vi "ContinuosSoundEntry.vi"() -> ()   [LabVIEW 2015]
uses:
  <vilib>/sound2/lvsound2.llb/Sound Data Format.ctl
  <vilib>/sound2/lvsound2.llb/Sampling Mode.ctl
  <vilib>/sound2/lvsound2.llb/Sound Input Read (DBL).vi
panel:
  out "data":waveform(dbl)[](array[waveform])
  out "Waveform Graph":waveform(dbl)[](graph)
  in  "stop":bool
  in  "sound format":T1={"sample rate (S/s)"=22050.0, "number of channels"=2, "bits per sample"=16}
  in  "device ID":u32
  in  "number of samples/ch":i32=100000
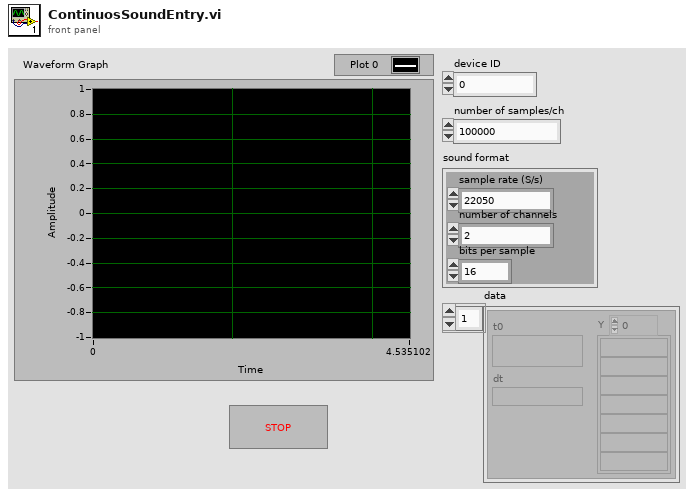
[diagram p1: front panel]
types:
  T1 = typedef "Sound Data Format.ctl" = cluster{"sample rate (S/s)":dbl, "number of channels":i32, "bits per sample":i32}
  T2 = typedef "Sampling Mode.ctl" = i32
  T3 = typedef "Sound Input Task ID.ctl" = u32
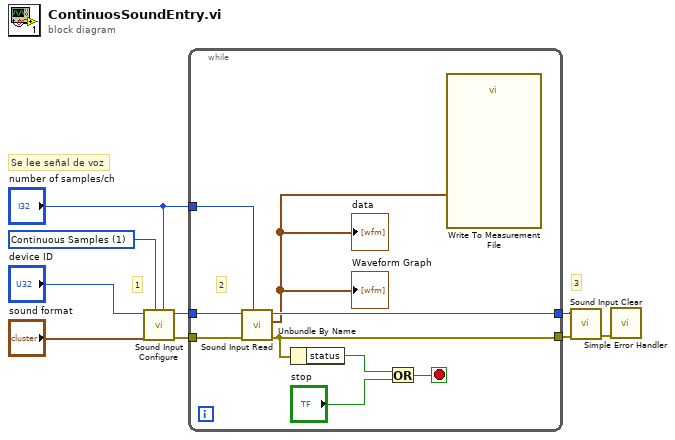
[diagram p0: block diagram]
diagram:
  w9 = T2 1 items=["Finite Samples", "Continuous Samples"] ("sample mode")
  # "3"
  # "1"
  # "Se lee señal de voz"
  n1 = call <vilib>:"Sound Input Configure.vi"("number of samples/ch"="number of samples/ch", "sample mode"=w9, "sound format"="sound format", "device ID"="device ID") -> ("error out"=w5:errorcluster, "task ID"=w6:T3)  [unwired: 6 in]
  n2 = while {
    tunnel: w6 -> [w18]
    tunnel: w5 -> [w17]
    tunnel: "number of samples/ch" -> [w16]
    tunnel: [w15] -> w3
    tunnel: [w14] -> w2
    stop <- w11 stop-if-true
    # "2"
    n3 = call-poly <vilib>:"Sound Input Read.vi"("number of samples/ch"=w16, "error in (no error)"=w17, "task ID"=w18) -> ("error out"=w14:errorcluster, "data"=w10:waveform(dbl)[], "task ID out"=w15:T3)  [unwired: 6 in]
    "Waveform Graph" <- w10
    "data" <- w10
    n4 = Unbundle By Name(w14) -> ("status"=w13:bool)
    n5 = Or(x=w13, y="stop") -> (x .or. y?=w11:bool)
    n6 = call "Write To Measurement File"("Signals"=w10) -> ()  [unwired: 16 in, 3 out]
  }
  n7 = call <vilib>:"Sound Input Clear.vi"("error in (no error)"=w2, "task ID"=w3) -> ("error out"=w1:errorcluster)  [unwired: 9 in]
  n8 = call <vilib>:"Simple Error Handler.vi"("error in (no error)"=w1) -> ()  [unwired: 4 in, 5 out]
